vi "FFT PtByPt.vi"   [LabVIEW 2020, in "NI_PtbyPt.lvlib"]
doc: "Computes the Fourier transform of <B>x</B>. This VI is similar to the FFT VI. Wire data to the <B>x</B> input to determine the polymorphic instance to use or manually select the instance."
uses:
  NI_PtbyPt.lvlib
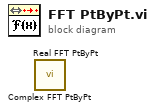
[diagram p0: block diagram]
diagram:
  n1 = call "Complex FFT PtByPt.vi"() -> ()  [unwired: 4 in, 2 out]
  n2 = call "Real FFT PtByPt.vi"() -> ()  [unwired: 4 in, 2 out]
